vi "Array To Set.vi"(11 "Array[]":string[](array[string])) -> (3 "Set":set{string}(c389))   [LabVIEW 2023, in "SLL Environment Variable.lvlib"]
doc: "Convert array to set"
uses:
  SLL Environment Variable.lvlib
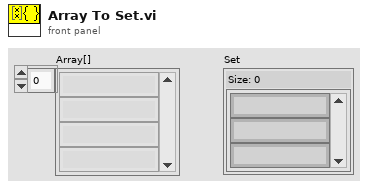
[diagram p1: front panel]
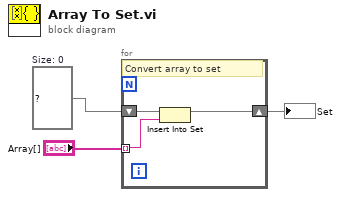
[diagram p0: block diagram]
diagram:
  w2 = set{string} {}  # Size: 0
  n1 = for {
    tunnel: "Array[]" -> [w5] mode=indexing
    shift-right: [w4] -> w1
    shift-left: w2 -> [w6]
    # "Convert array to set"
    n2 = Insert Into Set(10:w5, 11:w6) -> (3:w4:set{string})  [unwired: 1 out]
  }
  "Set" <- w1
